vi "Tosca-Start Pupillometry Recording.vi"(0 "Path":path, 11 "error in (no error)":errorcluster) -> (15 "error out":errorcluster)   [LabVIEW 2020]
uses:
  epl-vi-lib/TCP VIs/TCP Params.ctl
  epl-vi-lib/TCP VIs/TCP Write.vi
  Tosca-Globals.vi
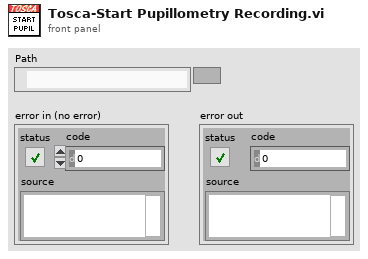
[diagram p1: front panel]
types:
  T1 = enum16{"big-endian, network order", "native, host order", "little-endian"}
  T2 = typedef "TCP Params.ctl" = cluster{"IP Address":string, "Port":i32}
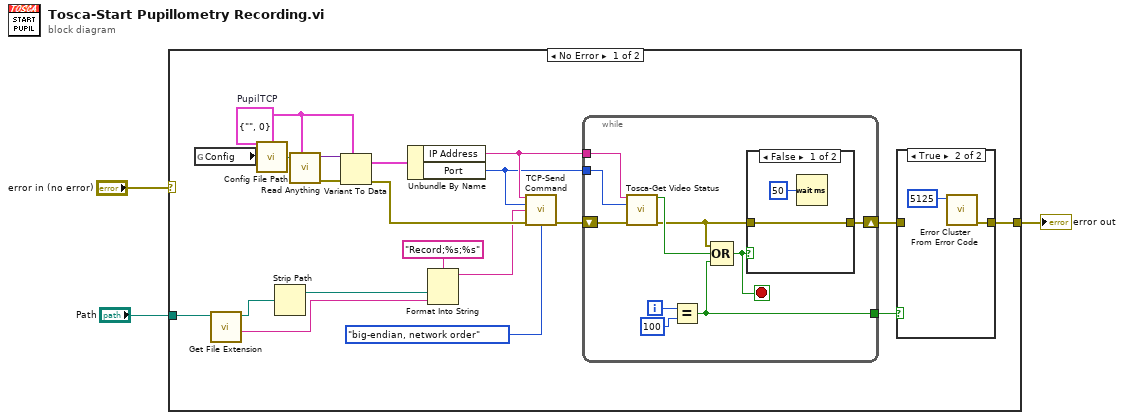
[diagram p0: block diagram]
diagram:
  n1 = case shown="No Error" "error in (no error)" {
    selector: "error in (no error)" -> [_ w40]
    tunnel: [w9 w40] -> w2
    tunnel: "Path" -> [w17 _]
    frame No Error {
      w22 = T2 {"IP Address"="", "Port"=0}  # PupilTCP
      n2 = global read "Tosca-Globals.vi" "Config"() -> (w5:string)
      n3 = call <vilib>:"Get File Extension.vi"("file"=w17) -> ("filename without extension"=w13:string, "dup file"=w15:path)  [unwired: 6 in, 3 out]
      n4 = call "Config File Path.vi"("AppName"=w5) -> ("Default config file name"=w23:path)
      n5 = Strip Path(path=w15) -> (stripped path=w14:path)  [unwired: 1 out]
      n6 = call "Read Anything.vi"("Type of Anything"=w22, "Path (dialog)"=w23) -> ("Error Out"=w20:errorcluster, "Anything"=w21:variant)  [unwired: 7 in, 1 out]
      n7 = Variant To Data(error in=w20, type=w22, Variant=w21) -> (data=w19:T2, error out=w18:errorcluster)
      n8 = Unbundle By Name(w19) -> ("IP Address"=w12:string, "Port"=w11:i32)
      n9 = Format Into String(format string="Record;%s;%s", w14, w13) -> (resulting string=w6:string)  [unwired: 2 in, 1 out]
      n10 = call "TCP-Send Command.vi"("PXI Address"=w12, "Port"=w11, "Command"=w6, "error in (no error)"=w18, "byte order"=T1."big-endian, network order") -> ("error out"=w10:errorcluster)  [unwired: 10 in]
      n11 = while {
        tunnel: w12 -> [w33]
        tunnel: w11 -> [w32]
        shift-right: [w28] -> w7
        shift-left: w10 -> [w31]
        tunnel: [w25] -> w8
        i -> [w27]
        stop <- w26 stop-if-true
        n12 = call "Tosca-Get Video Status.vi"("IP Address"=w33, "Port"=w32, "error in (no error)"=w31) -> ("Recording"=w30:bool, "error out"=w29:errorcluster)  [unwired: 11 in]
        n13 = Equal?(x=w27, y=100) -> (x = y?=w25:bool)
        n14 = Compound Arithmetic op=OR(w29, w30, w25) -> (w26:bool)
        n15 = case shown="False" w26 {
          tunnel: w29 -> [w34 w36]
          tunnel: [w34 w36] -> w28
          frame False {
            n16 = Wait (ms)(milliseconds to wait=u32 50) -> ()  [unwired: 1 out]
          }
          frame True {
          }
        }
      }
      n17 = case shown="True" w8 {
        tunnel: w7 -> [w37 _]
        tunnel: [w37 w39] -> w9
        frame False {
        }
        frame True {
          n18 = call <vilib>:"Error Cluster From Error Code.vi"("error code (0)"=5125) -> ("error out"=w39:errorcluster)  [unwired: 8 in]
        }
      }
    }
    frame Error {
    }
  }
  "error out" <- w2
